vi "Kaelus PIM Launch PIMHW Connection Daemon.vi"(8 "error in (no error)":errorcluster, 10 "port (3388)":u16=3388, 11 "PIMHW Host (\"localhost\")":string="localhost") -> (0 "error out":errorcluster)   [LabVIEW 2011]
uses:
  TypeDefs/PIMHW Connection CMDS.ctl
panel:
  in  "ConnectQ":string="PIMDaemonQ"
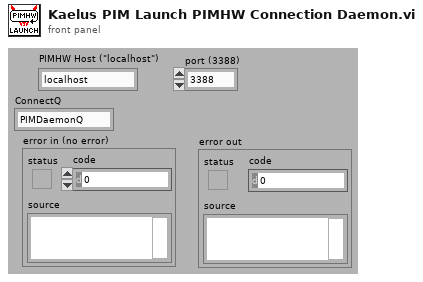
[diagram p1: front panel]
types:
  T1 = typedef "PIMHW Connection CMDS.ctl" = enum16{"CONNECT", "DISCONNECT", "KEEP_ALIVE"}
  T2 = enum32{"Bad", "Idle", "Run top level", "Running"}
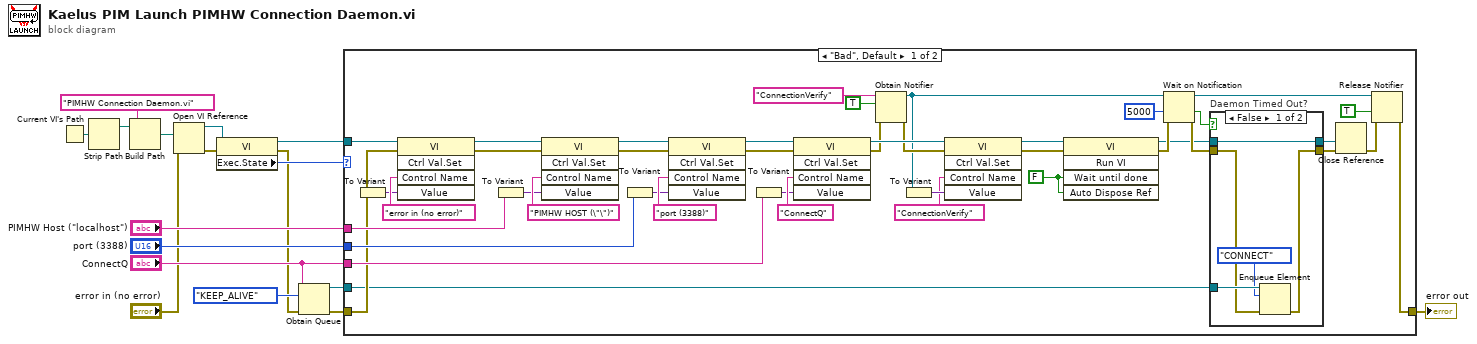
[diagram p0: block diagram]
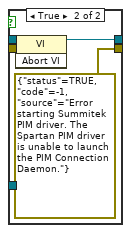
[diagram p2: hidden frame]
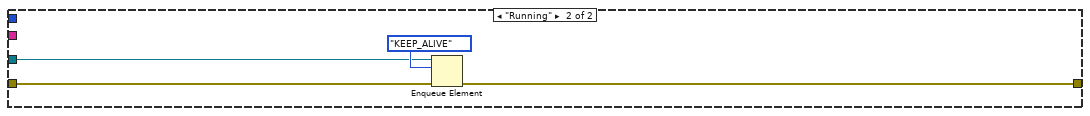
[diagram p3: hidden frame]
diagram:
  n1 = Current VI's Path() -> (path=w16:path)
  n2 = Strip Path(path=w16) -> (stripped path=w15:path)  [unwired: 1 out]
  n3 = Build Path(base path=w15, name or relative path="PIMHW Connection Daemon.vi") -> (appended path=w17:path)
  n4 = Open VI Reference(vi path=w17, error in (no error)="error in (no error)") -> (vi reference=w13:refnum<vi>, error out=w8:errorcluster)  [unwired: 4 out]
  n5 = property class="VI"(reference=w13, error in=w8) -> (reference out=w11:refnum<vi>, error out=w2:errorcluster, "Exec.State"=w12:T2)
  n6 = Obtain Queue(name (unnamed)="ConnectQ", element data type=PIMHW_Connection_CMDS."KEEP_ALIVE" ("Connection Commands"), error in (no error)=w2) -> (queue out=w5:refnum<queue>, error out=w4:errorcluster)  [unwired: 2 in, 1 out]
  n7 = case shown="\"Bad\", Default" w12 {
    tunnel: w11 -> [w59 _]
    tunnel: "PIMHW Host (\"localhost\")" -> [w52 _]
    tunnel: "port (3388)" -> [w49 _]
    tunnel: "ConnectQ" -> [w42 _]
    tunnel: w5 -> [w22 w71]
    tunnel: w4 -> [w41 w70]
    tunnel: [w23 w69] -> w1
    frame "Bad", Default {
      w29 = FALSE ("Wait Until Done")
      n8 = To Variant(anything=w41) -> (Variant=w57:variant)
      n9 = invoke class="VI" method="Ctrl Val.Set"(reference=w59, error in=w41, "Control Name"="error in (no error)", "Value"=w57) -> (reference out=w56:refnum<vi>, error out=w55:errorcluster)  [unwired: 1 in, 3 out]
      n10 = To Variant(anything=w52) -> (Variant=w53:variant)
      n11 = invoke class="VI" method="Ctrl Val.Set"(reference=w56, error in=w55, "Control Name"="PIMHW HOST (\"\")", "Value"=w53) -> (reference out=w47:refnum<vi>, error out=w48:errorcluster)  [unwired: 1 in, 3 out]
      n12 = To Variant(anything=w49) -> (Variant=w50:variant)
      n13 = invoke class="VI" method="Ctrl Val.Set"(reference=w47, error in=w48, "Control Name"="port (3388)", "Value"=w50) -> (reference out=w43:refnum<vi>, error out=w44:errorcluster)  [unwired: 1 in, 3 out]
      n14 = To Variant(anything=w42) -> (Variant=w45:variant)
      n15 = invoke class="VI" method="Ctrl Val.Set"(reference=w43, error in=w44, "Control Name"="ConnectQ", "Value"=w45) -> (reference out=w37:refnum<vi>, error out=w35:errorcluster)  [unwired: 1 in, 3 out]
      n16 = Obtain Notifier(name (unnamed)="ConnectionVerify", notification data type=TRUE ("Wait until done"), error in (no error)=w35) -> (notifier out=w33:refnum<notifier>, error out=w34:errorcluster)  [unwired: 1 in, 1 out]
      n17 = To Variant(anything=w33) -> (Variant=w38:variant)
      n18 = invoke class="VI" method="Ctrl Val.Set"(reference=w37, error in=w34, "Control Name"="ConnectionVerify", "Value"=w38) -> (reference out=w31:refnum<vi>, error out=w32:errorcluster)  [unwired: 1 in, 3 out]
      n19 = invoke class="VI" method="Run VI"(reference=w31, error in=w32, "Wait until done"=w29, "Auto Dispose Ref"=w29) -> (reference out=w21:refnum<vi>, error out=w30:errorcluster)  [unwired: 1 in, 3 out]
      n20 = Wait on Notification(notifier=w33, timeout in ms (-1)=5000, error in (no error)=w30) -> (notifier out=w24:refnum<notifier>, timed out?=w27:bool, error out=w26:errorcluster)  [unwired: 2 out]
      n21 = case "Daemon Timed Out?" shown="False" w27 {
        tunnel: w26 -> [w63 w68]
        tunnel: [w62 errorcluster {"status"=TRUE, "code"=-1, "source"="Error starting Summitek PIM driver. The Spartan PIM driver is unable to launch the PIM Connection Daemon."} ("error out")] -> w19
        tunnel: w22 -> [w64 _]
        tunnel: w21 -> [w60 w66]
        tunnel: [w60 w65] -> w20
        frame False {
          n22 = Enqueue Element(queue=w64, element=PIMHW_Connection_CMDS."CONNECT" ("Connection Commands"), error in (no error)=w63) -> (error out=w62:errorcluster)  [unwired: 1 in, 2 out]
        }
        frame True {
          n23 = invoke class="VI" method="Abort VI"(reference=w66, error in=w68) -> (reference out=w65:refnum<vi>)  [unwired: 1 in, 2 out]
        }
      }
      n24 = Close Reference(reference=w20, error in (no error)=w19) -> (error out=w18:errorcluster)
      n25 = Release Notifier(notifier=w24, force destroy? (F)=TRUE, error in (no error)=w18) -> (error out=w23:errorcluster)  [unwired: 2 out]
    }
    frame "Running" {
      n26 = Enqueue Element(queue=w71, element=PIMHW_Connection_CMDS."KEEP_ALIVE" ("Connection Commands"), error in (no error)=w70) -> (error out=w69:errorcluster)  [unwired: 1 in, 2 out]
    }
  }
  "error out" <- w1
